vi "清空列表.vi"(10 "列表":refnum<vi>) -> ()   [LabVIEW 2020]
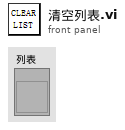
[diagram p1: front panel]
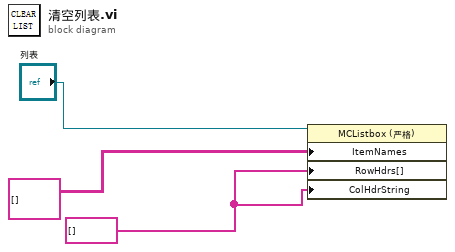
[diagram p0: block diagram]
diagram:
  w1 = string[] []
  n1 = property class="MCListbox (严格)"(reference="列表", "ItemNames"=string[][] [], "RowHdrs[]"=w1, "ColHdrString"=w1) -> ()  [unwired: 1 in, 2 out]
